vi "Get All Names and Values.vi"(8 "error in":errorcluster, 11 "Cluster In":variant) -> (0 "error out":errorcluster, 1 "Values":variant[](array[variant]), 2 "Item Names":string[](array[string]), 3 "Cluster Out":variant, 4 "Name":string)   [LabVIEW 2017, in "Advanced Variant Tools.lvlib" / "Cluster Manipulation.lvlib"]
doc: "Returns an array of all of the keys and an array of their corresponding values. Elements are correlated by index, so the key at a given index corresponds to the value at the same index."
uses:
  Cluster Manipulation.lvlib
  <vilib>/Utility/Data Type/NI_Data Type.lvlib
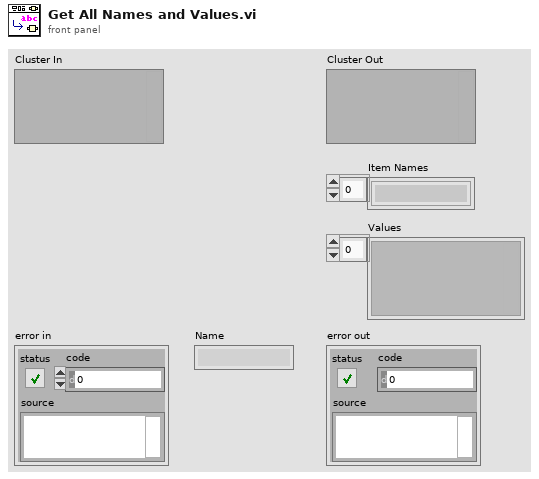
[diagram p1: front panel]
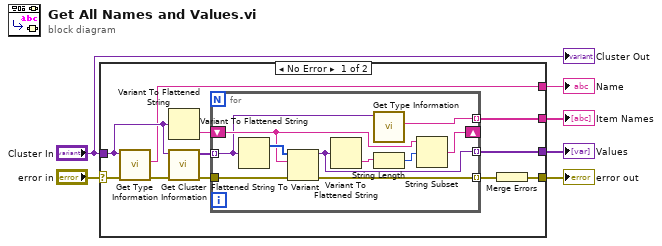
[diagram p0: block diagram]
diagram:
  n1 = case shown="No Error" "error in" {
    selector: "error in" -> [w13 w28]
    tunnel: "Cluster In" -> [w8 _]
    tunnel: [w12 w28] -> w4
    tunnel: [w11 _] -> w3
    tunnel: [w10 _] -> w2
    tunnel: [w7 _] -> w1
    frame No Error {
      n2 = call <vilib>:"Get Type Information.vi"("error in (no error)"=w13, "Variant"=w8) -> ("error out"=w9:errorcluster, "Name"=w7:string)  [unwired: 5 in, 3 out]
      n3 = Variant To Flattened String(Variant=w8) -> (data string=w14:string)  [unwired: 1 out]
      n4 = call <vilib>:"Get Cluster Information.vi"("error in (no error)"=w9, "Variant"=w8) -> ("error out"=w16:errorcluster, "Cluster Elements"=w15:variant[])  [unwired: 8 in]
      n5 = for {
        tunnel: w15 -> [w19] mode=indexing
        tunnel: [w26] -> w11 mode=indexing
        shift-right: [w22] -> _
        shift-left: w14 -> [w25]
        tunnel: w16 -> [w21]
        tunnel: [w20] -> w17 mode=indexing
        tunnel: [w18] -> w10 mode=indexing
        n6 = Variant To Flattened String(Variant=w19) -> (1:w27:i16[])  [unwired: 1 out]
        n7 = Flattened String To Variant(4:w21, 6:w25, 7:w27) -> (0:w20:errorcluster, 3:w26:variant)
        n8 = Variant To Flattened String(Variant=w26) -> (data string=w24:string)  [unwired: 1 out]
        n9 = call <vilib>:"Get Type Information.vi"("Variant"=w19) -> ("Name"=w18:string)  [unwired: 6 in, 4 out]
        n10 = String Length(string=w24) -> (length=w23:i32)
        n11 = String Subset(string=w25, offset (0)=w23) -> (substring=w22:string)  [unwired: 1 in]
      }
      n12 = Merge Errors(w17) -> (w12:errorcluster)
    }
    frame Error {
    }
  }
  "Item Names" <- w2
  "Values" <- w3
  "error out" <- w4
  "Name" <- w1
  "Cluster Out" <- "Cluster In"
